vi "Add Device Description Comments.vi"(7 "error in (no error)":errorcluster, 9 "Device Description":string, 10 "Comments in":string) -> (0 "error out":errorcluster, 3 "Comments":string)   [LabVIEW 2016, in "Control Experiment.lvclass"]
uses:
  Control Experiment.lvclass
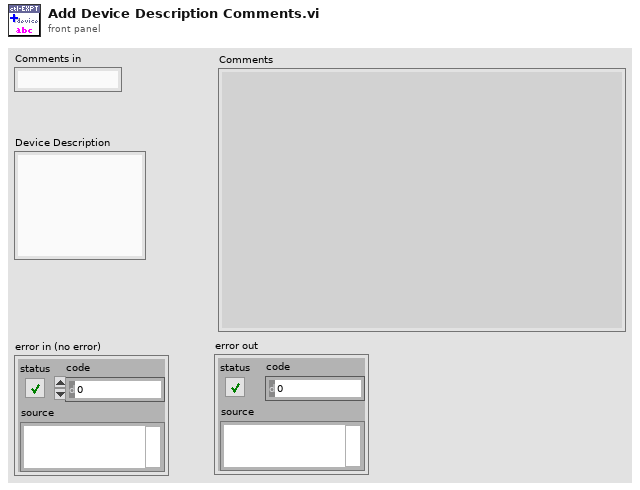
[diagram p1: front panel]
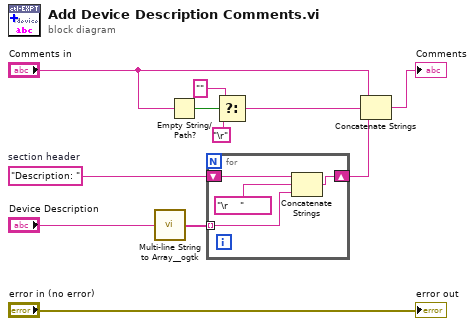
[diagram p0: block diagram]
diagram:
  w6 = "Description: "  # section header
  n1 = call <userlib>:"Multi-line String to Array__ogtk.vi"("string"="Device Description") -> ("lines"=w7:string[])
  n2 = Empty String/Path?(string/path="Comments in") -> (empty?=w10:bool)
  n3 = for {
    shift-right: [w15] -> w2
    shift-left: w6 -> [w14]
    tunnel: w7 -> [w12] mode=indexing
    n4 = Concatenate Strings(w14, "\r    " ("string"), w12) -> (w15:string)
  }
  n5 = Select(t="", s=w10, f="\r") -> (s? t:f=w3:string)
  n6 = Concatenate Strings("Comments in", w3, w2) -> (→"Comments":string)
  "error out" <- "error in (no error)"
